vi "Set Overlay Settings.vi"(8 "error in (no error)":errorcluster, 10 "Overlay Settings":refnum<class "Analyze Results Base.lvclass">[](array[class]), 11 "HIJ Vision Display in":refnum<class "HIJ Vision Display.lvclass">) -> (0 "error out":errorcluster, 3 "HIJ Vision Display out":refnum<class "HIJ Vision Display.lvclass">)   [LabVIEW 2014, in "HIJ Vision Display.lvlib" / "HIJ Vision Display.lvclass"]
uses:
  HIJ Vision Display.lvclass
  Results and Overlays/Results Base/Analyze Results Base.lvclass
  HIJ Vision Display.lvclass/HIJ Vision Display.ctl
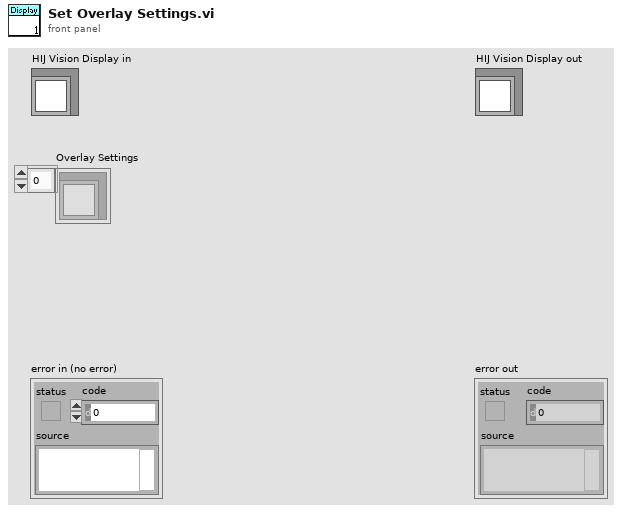
[diagram p1: front panel]
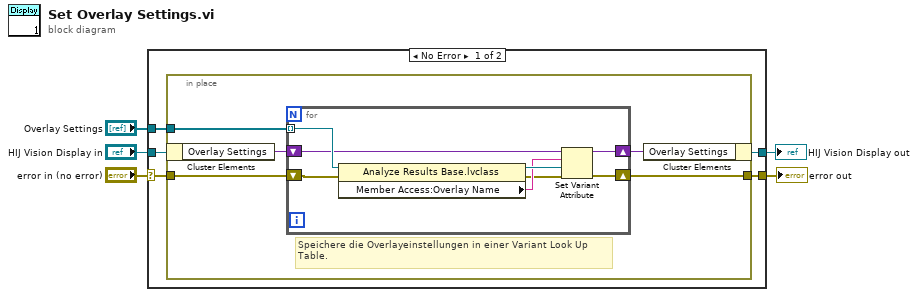
[diagram p0: block diagram]
diagram:
  n1 = case shown="No Error" "error in (no error)" {
    selector: "error in (no error)" -> [w8 w25]
    tunnel: [w7 w25] -> w4
    tunnel: [w6 w24] -> w2
    tunnel: "HIJ Vision Display in" -> [w9 w24]
    tunnel: "Overlay Settings" -> [w10 _]
    frame No Error {
      n2 = in-place {
        in-place-border: w10 -> [w15]
        in-place-border: w8 -> [w13]
        in-place-border: [w12] -> w7
        # "Speichere die Overlayeinstellungen in einer Variant Look Up\nTable."
        n3 = in-place-cluster #1(w9) -> ("Overlay Settings"=w14:variant)
        n4 = for {
          tunnel: w15 -> [w23] mode=indexing
          shift-right: [w21] -> w12
          shift-left: w13 -> [w17]
          shift-right: [w20] -> w11
          shift-left: w14 -> [w22]
          n5 = property class="Analyze Results Base.lvclass"(reference=w23, error in=w17) -> (reference out=w19:refnum<class "Analyze Results Base.lvclass">, error out=w16:errorcluster, "Member Access:Overlay Name"=w18:string)
          n6 = Set Variant Attribute(Variant=w22, name=w18, value=w19, error in=w16) -> (Variant out=w20:variant, error out=w21:errorcluster)  [unwired: 1 out]
        }
        n7 = in-place-cluster #1("Overlay Settings"=w11) -> (w6:refnum<class "HIJ Vision Display.lvclass">)
      }
    }
    frame Error {
    }
  }
  "error out" <- w4
  "HIJ Vision Display out" <- w2
